vi "Build Module v2.vi"() -> ()   [LabVIEW 2016]
uses:
  Status.vi
  Classes/Assembly/Assembly Run.lvclass
  Classes/Controller/Controller.lvclass
  Classes/Module/Module.lvclass
  Classes/Routine/Settings.ctl
  Classes/Routine/Routine.lvclass
panel:
  in  "Number of Modules":i32
  in  "Run":bool
  in  "Glue step":enum16{"Kapton", "Sensor", "PCB"}(ring)
  in  "Add":bool
  in  "Number of modules":i32
  in  "Baseplate Tray ID":i32
  out "Status":T1
  in  "Open I/O Test":bool
  in  "Stop":bool
  # "Region 3"
  # "Region 2"
  # "Region 1"
  # "Position 2"
  # "Position 1"
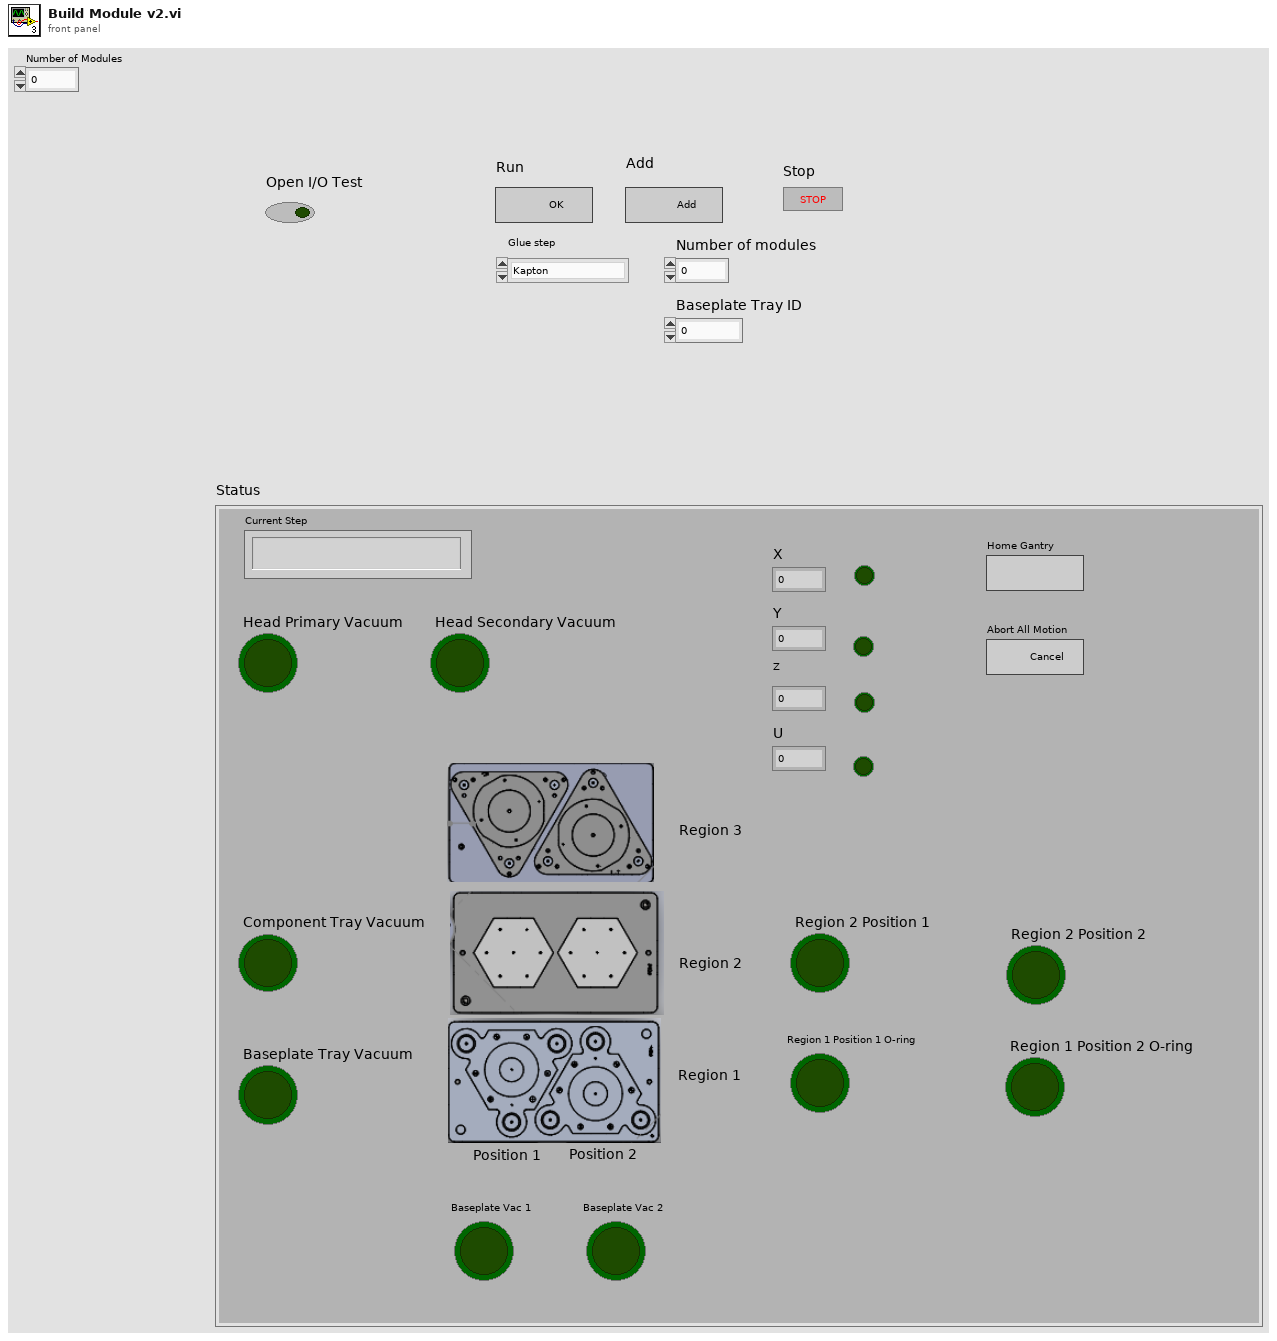
[diagram p1: front panel]
types:
  T1 = cluster{"Current Step":string, "Baseplate Tray Vacuum":bool, "Component Tray Vacuum":bool, "Head Primary Vacuum":bool, "Head Secondary Vacuum":bool, "Region 1 Position 1 O-ring":bool, "Region 1 Position 2 O-ring":bool, "Region 2 Position 1":bool, "Region 2 Position 2":bool, "X":dbl, "Y":dbl, "Z":dbl, "U":dbl, "Home Gantry":bool, bool, bool, bool, bool, "Abort All Motion":bool, "Baseplate Vac 1":bool, "Baseplate Vac 2":bool}
  T2 = enum32{"Invalid", "Standard", "Closed", "Hidden", "Minimized", "Maximized"}
  T3 = typedef "Routine.lvclass/Settings.ctl" = enum16{"Default", "Custom"}
  T4 = cluster{"Current Step":string, "Baseplate Tray Vacuum":bool, "Component Tray Vacuum":bool, "Head Primary Vacuum":bool, "Head Secondary Vacuum":bool, "Region 1 Position 1 O-ring":bool, "Region 1 Position 2 O-ring":bool, "Region 2 Position 1":bool, "Region 2 Position 2":bool, "X":dbl, "Y":dbl, "Z":dbl, "U":dbl, "Home Position":bool, "Enabled":bool, "Enabled 2":bool, bool, bool, "Abort All Motion":bool, "Baseplate Vac 1":bool, "Baseplate Vac 2":bool}
  T5 = typedef "Controller.lvclass/Controllers.ctl" = cluster{"I-O.lvclass":refnum<class "I-O.lvclass">, "Motion.lvclass":refnum<class "Motion.lvclass">, "Dispenser.lvclass":refnum<class "Dispenser.lvclass">}
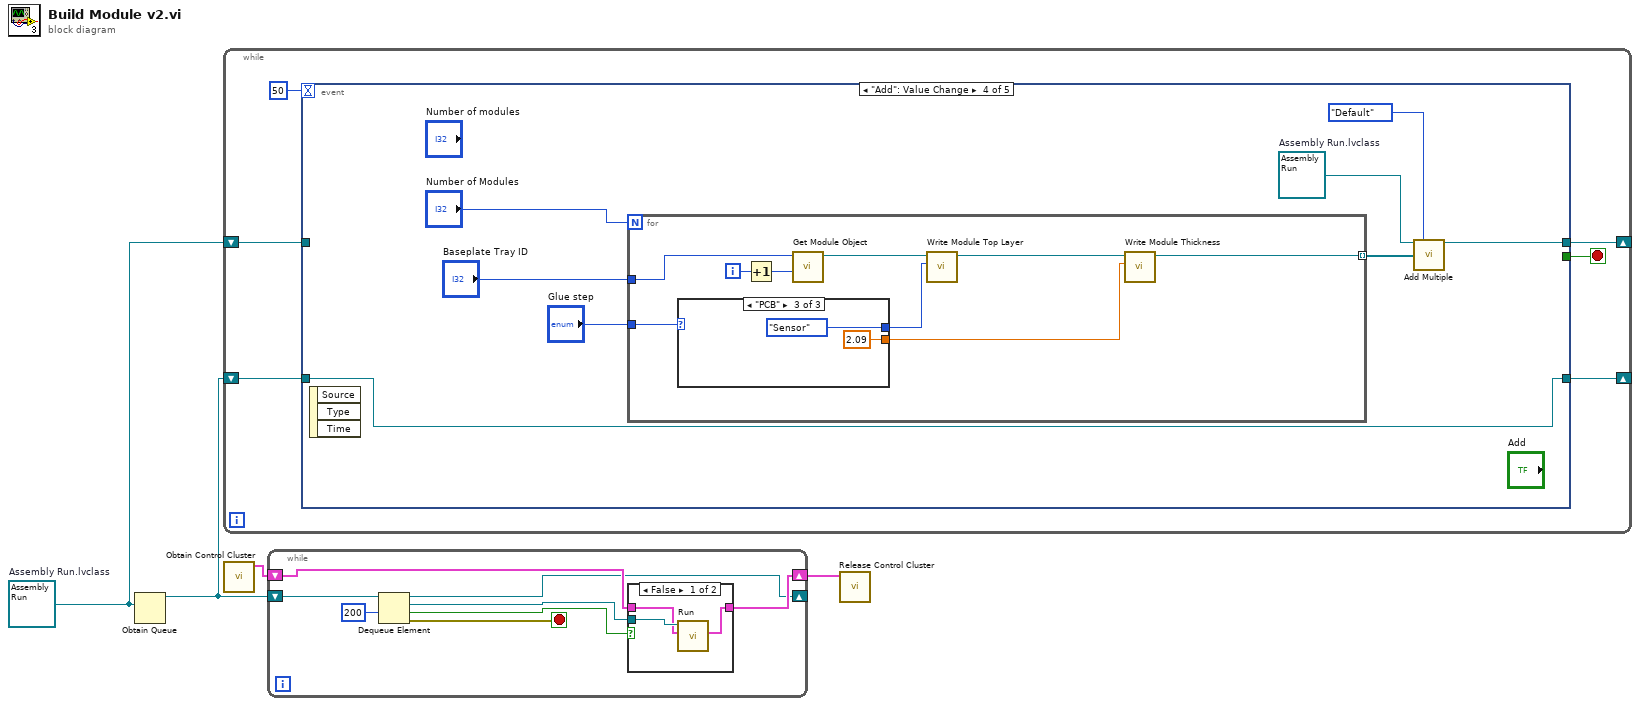
[diagram p0: block diagram]
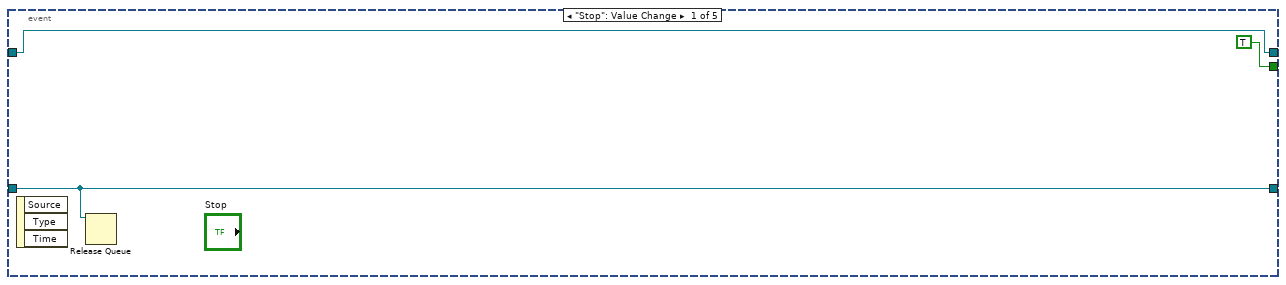
[diagram p3: hidden frame]
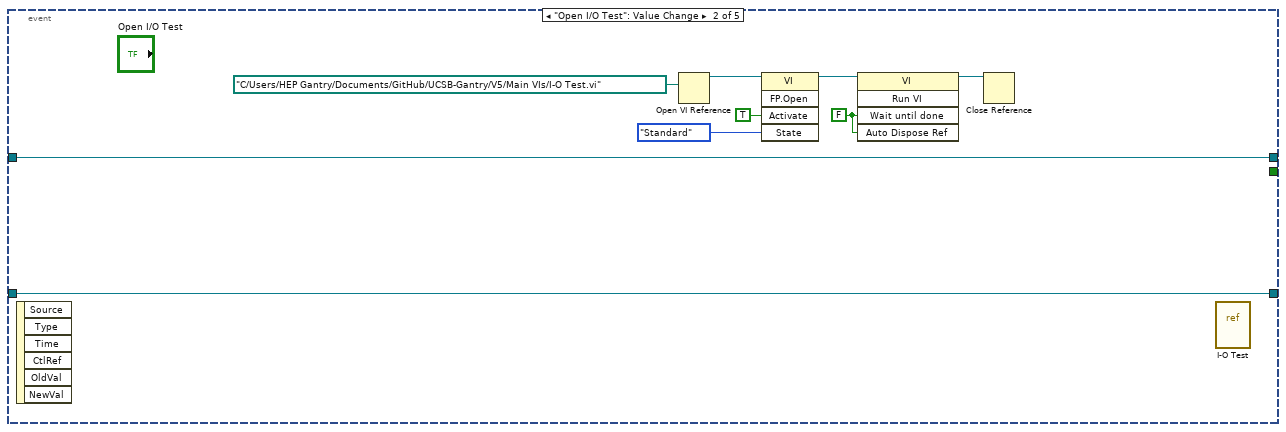
[diagram p4: hidden frame]
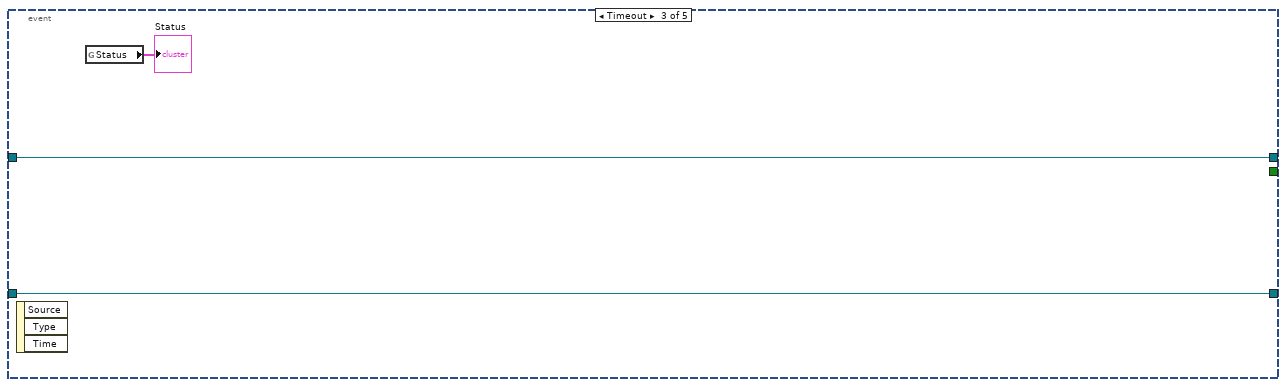
[diagram p5: hidden frame]
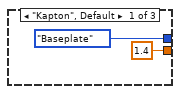
[diagram p6: hidden frame]
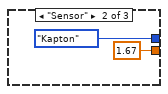
[diagram p7: hidden frame]
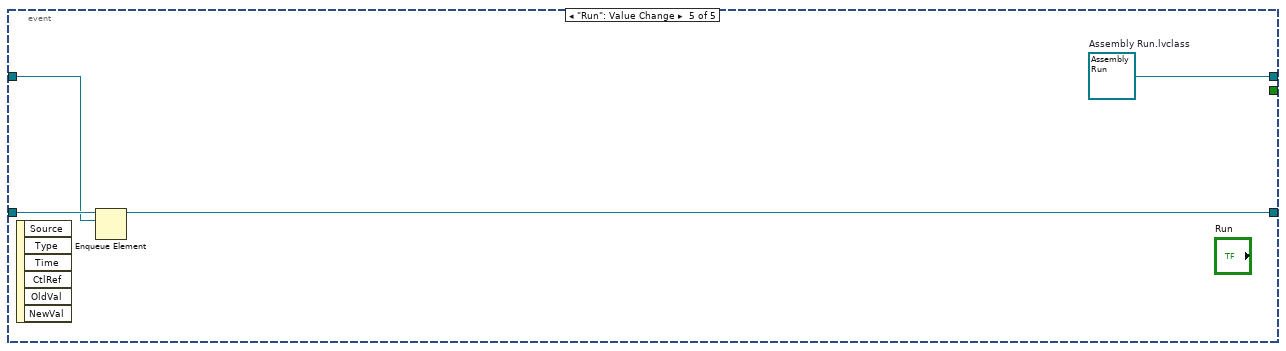
[diagram p8: hidden frame]
diagram:
  w1 = refnum<class "Assembly Run.lvclass"> refnum  # Assembly Run.lvclass
  n1 = Obtain Queue(element data type=w1) -> (queue out=w4:refnum<queue>)  [unwired: 4 in, 2 out]
  n2 = while {
    shift-right: [w9] -> _
    shift-left: w4 -> [w10]
    shift-right: [w7] -> _
    shift-left: w1 -> [w6]
    stop <- w8 stop-if-true
    n3 = event shown="[3] \"Add\": Value Change" {
      selector: _ -> [_ _ _ _ _]
      dyn-events: _ -> [_ _ _ _ _]
      timeout: 50 -> [_ _ _ _ _]
      tunnel: w10 -> [w11 w20 w24 w33 w51]
      tunnel: [w11 w20 w24 w33 w49] -> w9
      tunnel: [TRUE _ _ _ _] -> w8
      tunnel: [w12 w21 w25 w27 w52] -> w7
      tunnel: w6 -> [w12 w21 w25 _ w50]
      event "Stop": Value Change {
        n4 = event-data() -> ()  [unwired: 1 in, 3 out]
        n5 = Release Queue(queue=w11) -> ()  [unwired: 2 in, 3 out]
      }
      event "Open I/O Test": Value Change {
        w15 = FALSE
        n6 = event-data() -> ()  [unwired: 1 in, 6 out]
        n7 = Open VI Reference(vi path=path "C:/Users/HEP Gantry/Documents/GitHub/UCSB-Gantry/V5/Main VIs/I-O Test.vi") -> (vi reference=w19:refnum<vi>)  [unwired: 5 in, 1 out]
        n8 = invoke class="VI" method="FP.Open"(reference=w19, "Activate"=TRUE, "State"=T2."Standard") -> (reference out=w16:refnum<vi>)  [unwired: 2 in, 4 out]
        n9 = invoke class="VI" method="Run VI"(reference=w16, "Wait until done"=w15, "Auto Dispose Ref"=w15) -> (reference out=w14:refnum<vi>)  [unwired: 2 in, 4 out]
        n10 = Close Reference(reference=w14) -> ()  [unwired: 1 in, 1 out]
        n11 = vi-ref "I-O Test.vi"() -> ()  [unwired: 1 out]
      }
      event Timeout {
        n12 = event-data() -> ()  [unwired: 1 in, 3 out]
        n13 = global read "Status.vi" "Status"() -> (→"Status":T4)
      }
      event "Add": Value Change {
        w29 = refnum<class "Assembly Run.lvclass"> refnum  # Assembly Run.lvclass
        n14 = event-data() -> ()  [unwired: 1 in, 3 out]
        n15 = for {
          N: "Number of Modules" -> [_]
          tunnel: "Baseplate Tray ID" -> [w42]
          tunnel: [w35] -> w28 mode=indexing
          tunnel: "Glue step" -> [w38]
          i -> [w41]
          n16 = case shown="\"PCB\"" w38 {
            tunnel: [enum16{"Baseplate", "Kapton", "Sensor", "PCB"}."Baseplate" ("Module Top Layer") enum16{"Baseplate", "Kapton", "Sensor", "PCB"}."Kapton" ("Module Top Layer") enum16{"Baseplate", "Kapton", "Sensor", "PCB"}."Sensor" ("Module Top Layer")] -> w37
            tunnel: [1.4 1.67 2.09] -> w34
            frame "Kapton", Default {
            }
            frame "Sensor" {
            }
            frame "PCB" {
            }
          }
          n17 = Increment(x=w41) -> (x+1=w40:i32)
          n18 = call "Get Module Object.vi"("Assembly Tray Position"=w40, "Assembly Tray Number"=w42) -> ("Module.lvclass"=w39:refnum<class "Module.lvclass">)  [unwired: 8 in, 1 out]
          n19 = call "Write Module Top Layer.vi"("Module Top Layer"=w37, "Module in"=w39) -> ("Module out"=w36:refnum<class "Module.lvclass">)  [unwired: 8 in, 1 out]
          n20 = call-dynamic "Write Module Thickness.vi"("Module Thickness"=w34, "Module in"=w36) -> ("Module out"=w35:refnum<class "Module.lvclass">)  [unwired: 8 in, 1 out]
        }
        n21 = call-dynamic "Add Multiple.vi"("Assembly in"=w29, "Settings"=Settings."Default", "Modules"=w28) -> ("Assembly out"=w27:refnum<class "Assembly Run.lvclass">)  [unwired: 11 in, 1 out]
      }
      event "Run": Value Change {
        w52 = refnum<class "Assembly Run.lvclass"> refnum  # Assembly Run.lvclass
        n22 = event-data() -> ()  [unwired: 1 in, 6 out]
        n23 = Enqueue Element(queue=w51, element=w50) -> (queue out=w49:refnum<queue>)  [unwired: 2 in, 2 out]
      }
    }
  }
  n24 = call "Obtain Control Cluster.vi"() -> ("Control Out"=w2:T5)  [unwired: 11 in]
  n25 = while {
    shift-right: [w53] -> _
    shift-left: w4 -> [w60]
    shift-right: [w55] -> w3
    shift-left: w2 -> [w56]
    stop <- w54 stop-if-true
    n26 = Dequeue Element(queue=w60, timeout in ms (-1)=200) -> (queue out=w53:refnum<queue>, element=w59:refnum<class "Assembly Run.lvclass">, timed out?=w58:bool, error out=w54:errorcluster)  [unwired: 1 in]
    n27 = case shown="False" w58 {
      tunnel: w59 -> [w63 _]
      tunnel: w56 -> [w62 w64]
      tunnel: [w61 w64] -> w55
      frame False {
        n28 = call-dynamic "Run.vi"("Control In"=w62, "Assembly In"=w63) -> ("Control Out"=w61:T5)  [unwired: 7 in, 2 out]
      }
      frame True {
      }
    }
  }
  n29 = call "Release Control Cluster.vi"("output cluster"=w3) -> ()  [unwired: 11 in]
